vi "FP Origin.vi"(1 "vi path":path) -> (0 "error out":errorcluster)   [LabVIEW 2015]
uses:
  <vilib>/Utility/miscctls.llb/LVPointTypeDef.ctl
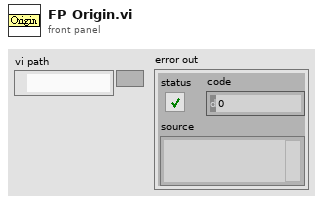
[diagram p1: front panel]
types:
  T1 = typedef "LVPointTypeDef.ctl" = cluster{"Horizontal":i16, "Vertical":i16}
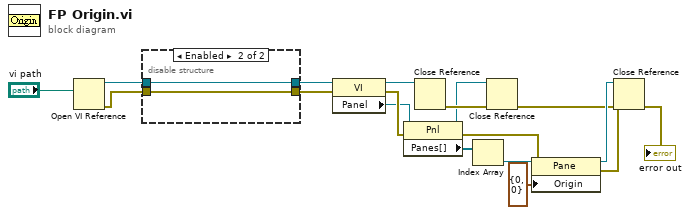
[diagram p0: block diagram]
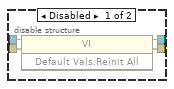
[diagram p2: hidden frame]
diagram:
  n1 = Open VI Reference(vi path="vi path") -> (vi reference=w5:refnum<vi>, error out=w3:errorcluster)  [unwired: 5 in]
  n2 = disable-structure shown="Enabled" {
    disable-tunnel: w5 -> [w21 w23]
    disable-tunnel: [w20 w23] -> w4
    disable-tunnel: w3 -> [w19 w22]
    disable-tunnel: [w18 w22] -> w2
    frame Disabled {
      n3 = invoke class="VI" method="Default Vals.Reinit All"(reference=w21, error in=w19) -> (reference out=w20:refnum<vi>, error out=w18:errorcluster)  [unwired: 1 in, 1 out]
    }
    frame Enabled {
    }
  }
  n4 = property class="VI"(reference=w4, error in=w2) -> (reference out=w7:refnum<vi>, error out=w14:errorcluster, "Panel"=w8:refnum<vi>)
  n5 = property class="Pnl"(reference=w8, error in=w14) -> (reference out=w12:refnum<vi>, error out=w15:errorcluster, "Panes[]"=w9:refnum<vi>[])
  n6 = Index Array(array=w9) -> (element=w10:refnum<vi>)  [unwired: 1 in]
  n7 = property class="Pane"(reference=w10, error in=w15, "Origin"=T1 {"Horizontal"=0, "Vertical"=0}) -> (reference out=w13:refnum<vi>, error out=w16:errorcluster)
  n8 = Close Reference(reference=w13, error in (no error)=w16) -> (error out=w1:errorcluster)
  "error out" <- w1
  n9 = Close Reference(reference=w12, error in (no error)=w1) -> (error out=w17:errorcluster)
  n10 = Close Reference(reference=w7, error in (no error)=w17) -> ()  [unwired: 1 out]
